vi "Log Event.vi"(6 "Event Time":timestamp, 7 "Event Level":T1, 8 "error in (no error)":errorcluster, 9 "Data To Log":string, 10 "SourceID":string, 11 "Log Instance":refnum<class "LoggerReference.lvclass">) -> (0 "error out":errorcluster, 3 "Log Instance Out":refnum<class "LoggerReference.lvclass">)   [LabVIEW 2020, in "Composed Log.lvlib" / "LoggerReference.lvclass"]
doc: "Write an event to the logger. This event will be captured by any active, sinks that have a defined log level at or below the event level."
uses:
  <vilib>/gpm_packages/@cs/event-logger/Source/Composed Log/LoggerReference/LoggerReference.lvclass
  <vilib>/gpm_packages/@cs/event-logger/Source/Composed Log/Types/Log Level.ctl
  <vilib>/gpm_packages/@cs/event-logger/Source/Composed Log/LoggerReference/LoggerReference.lvclass/LoggerReference.ctl
  <vilib>/gpm_packages/@cs/event-logger/Source/Composed Log/Types/Log Packet.ctl
  <vilib>/gpm_packages/@cs/event-logger/Source/Composed Log/LoggerReference/Remove Stale Logs.vi
  <vilib>/gpm_packages/@cs/event-logger/Source/Composed Log/Composed Log.lvlib
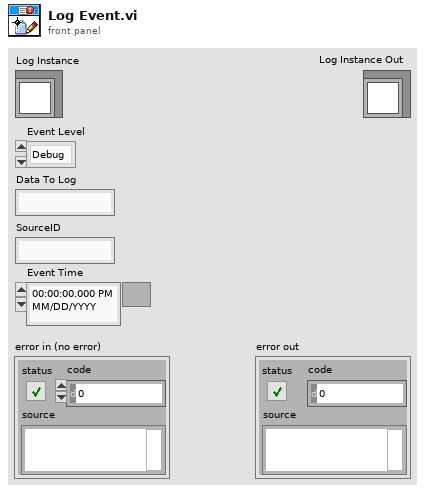
[diagram p1: front panel]
types:
  T1 = typedef "Composed Log.lvlib/Log Level.ctl" = enum16{"Debug", "Info", "Warning", "Error", "Critical"}
  T2 = typedef "Composed Log.lvlib/Log Packet.ctl" = cluster{"Data To Log":string, "Source":string, "Event Level":T1, "Event Time":timestamp}
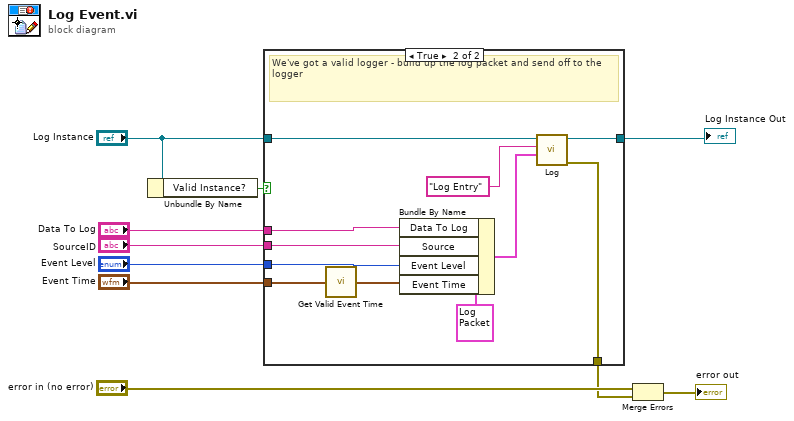
[diagram p0: block diagram]
diagram:
  n1 = Unbundle By Name("Log Instance") -> ("Valid Instance?"=w1:bool)
  n2 = case shown="True" w1 {
    tunnel: "Data To Log" -> [_ w21]
    tunnel: "Event Level" -> [_ w20]
    tunnel: "Event Time" -> [_ w13]
    tunnel: "SourceID" -> [_ w19]
    tunnel: [w11 w18] -> w3
    tunnel: [_ w17] -> w2
    tunnel: "Log Instance" -> [w11 w16]
    frame False {
      # "Not a valid instance of the logger - it was never initialized so do nothing - not returning an error was an intentional design decision to allow unit testing modules that call the logger"
    }
    frame True {
      # "We've got a valid logger - build up the log packet and send off to the logger"
      n3 = call <vilib>:"Get Valid Event Time.vi"("Event Time In"=w13) -> ("Event Time Out"=w12:timestamp)
      n4 = Bundle By Name(cluster=T2 {"Data To Log"="", "Source"="", "Event Level"=enum."Debug", "Event Time"=timestamp(0 s since 1904-01-01)} ("Log Packet"), "Data To Log"=w21, "Source"=w19, "Event Level"=w20, "Event Time"=w12) -> (w14:T2)
      n5 = call <vilib>:"Log.vi"("Log Packet"=w14, "Message"="Log Entry", "LoggerReference in"=w16) -> ("error out"=w17:errorcluster, "LoggerReference out"=w18:refnum<class "LoggerReference.lvclass">)  [unwired: 7 in]
    }
  }
  "Log Instance Out" <- w3
  n6 = Merge Errors("error in (no error)", w2) -> (→"error out":errorcluster)
